vi "PH_Sound.Ice Hockey 2.vi"() -> (0 "Ice Hockey 2":cluster{"Tone":dbl, "Beats":i32}[](array[cluster]))   [LabVIEW 2014, in "PH_Sound.lvlib"]
doc: "\"Alle Vögel sind schon da, ...\""
uses:
  PH_Sound.lvlib
  PH_Sound.3Oktaves.ctl
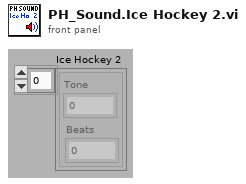
[diagram p1: front panel]
types:
  T1 = typedef "PH_Sound.lvlib/PH_Sound.3Oktaves.ctl" = dbl
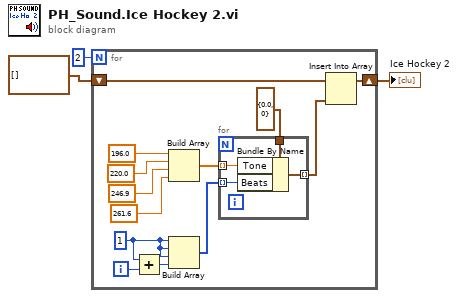
[diagram p0: block diagram]
diagram:
  n1 = for {
    N: 2 -> [_]
    shift-right: [w9] -> w3
    shift-left: cluster{"Tone":dbl, "Beats":i32}[] [] -> [w10]
    i -> [w6]
    w7 = u32 1 ("y")
    w12 = T1 261.6 items=["c"=130.8, "cis"=138.6, "d"=146.8, "es"=155.6, "e"=164.8, "f"=174.6, "fis"=185.0, "g"=196.0, "as"=207.6, "a"=220.0, "b"=233.1, "h"=246.9, "c'"=261.6, "cis'"=277.2, "d'"=293.7, "es'"=311.1, "e'"=329.6, "f'"=349.2, "fis'"=370.0, "g'"=392.0, "as'"=415.3, "a'"=440.0, "b'"=466.2, "h'"=493.9, "c''"=523.3, "cis''"=554.4, "d''"=587.3, "es''"=622.3, "e''"=659.3, "f''"=689.5, "fis''"=740.0, "g''"=784.0, "as''"=830.6, "a''"=880.0, "b''"=932.3, "h''"=987.8, "c'''"=1047.0] ("3 Octaves")
    w13 = T1 246.9 items=["c"=130.8, "cis"=138.6, "d"=146.8, "es"=155.6, "e"=164.8, "f"=174.6, "fis"=185.0, "g"=196.0, "as"=207.6, "a"=220.0, "b"=233.1, "h"=246.9, "c'"=261.6, "cis'"=277.2, "d'"=293.7, "es'"=311.1, "e'"=329.6, "f'"=349.2, "fis'"=370.0, "g'"=392.0, "as'"=415.3, "a'"=440.0, "b'"=466.2, "h'"=493.9, "c''"=523.3, "cis''"=554.4, "d''"=587.3, "es''"=622.3, "e''"=659.3, "f''"=689.5, "fis''"=740.0, "g''"=784.0, "as''"=830.6, "a''"=880.0, "b''"=932.3, "h''"=987.8, "c'''"=1047.0] ("3 Octaves")
    w15 = T1 220.0 items=["c"=130.8, "cis"=138.6, "d"=146.8, "es"=155.6, "e"=164.8, "f"=174.6, "fis"=185.0, "g"=196.0, "as"=207.6, "a"=220.0, "b"=233.1, "h"=246.9, "c'"=261.6, "cis'"=277.2, "d'"=293.7, "es'"=311.1, "e'"=329.6, "f'"=349.2, "fis'"=370.0, "g'"=392.0, "as'"=415.3, "a'"=440.0, "b'"=466.2, "h'"=493.9, "c''"=523.3, "cis''"=554.4, "d''"=587.3, "es''"=622.3, "e''"=659.3, "f''"=689.5, "fis''"=740.0, "g''"=784.0, "as''"=830.6, "a''"=880.0, "b''"=932.3, "h''"=987.8, "c'''"=1047.0] ("3 Octaves")
    w16 = T1 196.0 items=["c"=130.8, "cis"=138.6, "d"=146.8, "es"=155.6, "e"=164.8, "f"=174.6, "fis"=185.0, "g"=196.0, "as"=207.6, "a"=220.0, "b"=233.1, "h"=246.9, "c'"=261.6, "cis'"=277.2, "d'"=293.7, "es'"=311.1, "e'"=329.6, "f'"=349.2, "fis'"=370.0, "g'"=392.0, "as'"=415.3, "a'"=440.0, "b'"=466.2, "h'"=493.9, "c''"=523.3, "cis''"=554.4, "d''"=587.3, "es''"=622.3, "e''"=659.3, "f''"=689.5, "fis''"=740.0, "g''"=784.0, "as''"=830.6, "a''"=880.0, "b''"=932.3, "h''"=987.8, "c'''"=1047.0] ("3 Octaves")
    n2 = Add(x=w7, y=w6) -> (x+y=w5:u32)
    n3 = Build Array(w16, w15, w13, w12) -> (w14:T1[])
    n4 = Build Array(w7, w7, w7, w5) -> (w4:u32[])
    n5 = for {
      tunnel: w14 -> [w19] mode=indexing
      tunnel: cluster{"Tone":dbl, "Beats":i32} {"Tone"=0.0, "Beats"=0} ("Note") -> [w20]
      tunnel: [w18] -> w8 mode=indexing
      tunnel: w4 -> [w17] mode=indexing
      n6 = Bundle By Name(cluster=w20, "Tone"=w19, "Beats"=w17) -> (w18:cluster{"Tone":dbl, "Beats":i32})
    }
    n7 = Insert Into Array(array=w10, new element=w8) -> (w9:cluster{"Tone":dbl, "Beats":i32}[])  [unwired: 1 in]
  }
  "Ice Hockey 2" <- w3
